vi "ElevatorSystem.vi"(5 "Motor Output":dbl, 7 "Controller Override?":bool, 8 "Scoring Deploy Status":cluster{"State":enum16{"Idle", "Deploy"}}, 9 "Scoring Heights":i32[](array[numeric]), 10 "Device Names":string[](array[string]), 11 "Intake Status":T2) -> (3 "Elevator Status":T1)   [LabVIEW 2014]
panel:
  # "Proximity Sensor"
  # "Elevator Encoder"
  # "Elevator Motor"
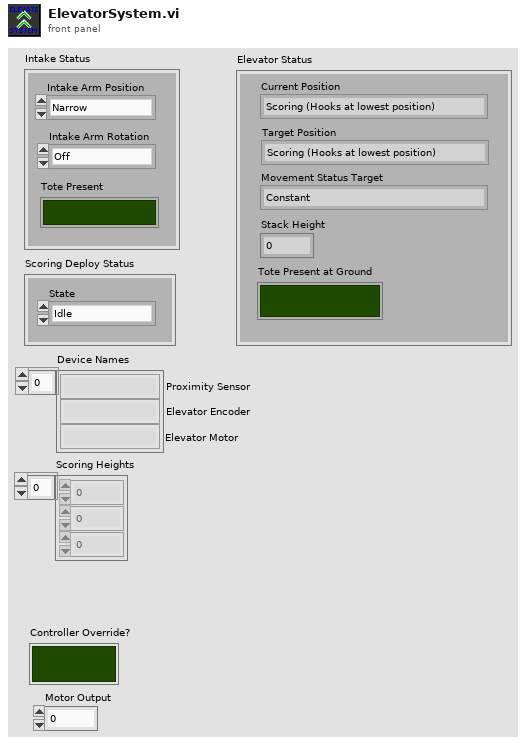
[diagram p1: front panel]
types:
  T1 = cluster{"Current Position":enum16{"Scoring (Hooks at lowest position)", "Intermediary (Between positions)", "Low (Hooks rest under lip)", "High (Holding totes up)"}, "Movement Status Target":enum16{"Constant", "Lifting", "Lowering"}, "Stack Height":i32, "Tote Present at Ground":bool, "Target Position":enum16{"Scoring (Hooks at lowest position)", "Low (Hooks rest under lip)", "High (Holding totes up)"}}
  T2 = cluster{"Intake Arm Position":enum16{"Narrow", "Wide"}, "Intake Arm Rotation":enum16{"Off", "In", "Out", "Rotate Tote"}, "Tote Present":bool}
  T3 = typedef "WPI_MotorControlDeviceRef.ctl" = cluster{"DeviceStatus":errorcluster, "Type":T4, "PWM":cluster{"Controller":T5, "PWM Channel":T6, "DeadBand":T7}, "CAN":cluster{"Device Number":u8, "Control Mode":T8, "Semaphore":T9, "Max Vout":dbl, "TalonSRX Control Mode":T10}, "Invert":bool, "TransformRef":T11, "InvTransformRef":T11}
  T4 = typedef "WPI_MotorControlType.ctl" = enum16{"PWM", "CAN", "CANTalonSRX"}
  T5 = typedef "FPGA_TypedefDigitalModule.ctl" = enum16{"Controller 1"}
  T6 = typedef "FPGA_DIOPWMChannel.ctl" = enum8{"PWM 0", "PWM 1", "PWM 2", "PWM 3", "PWM 4", "PWM 5", "PWM 6", "PWM 7", "PWM 8", "PWM 9", "PWM MXP 0", "PWM MXP 1", "PWM MXP 2", "PWM MXP 3", "PWM MXP 4", "PWM MXP 5", "PWM MXP 6", "PWM MXP 7", "PWM MXP 8", "PWM MXP 9", "Invalid"}
  T7 = typedef "WPI_PWMDeadband.ctl" = cluster{"Name":string, "maxPositivePwm":i32, "minPositivePwm":i32, "centerPwm":i32, "maxNegativePwm":i32, "minNegativePwm":i32, "angularRange":u16}
  T8 = typedef "WPI_CANJaguar_ControlMode.ctl" = enum8{"Percent VBus", "Current", "Speed", "Position", "Voltage"}
  T9 = typedef "Semaphore RefNum" = refnum<k1>
  T10 = typedef "WPI_CANTalonSRX_APIControlMode.ctl" = enum8{"Percent VBus", "Speed", "Position", "Slave", "Unchanged / Invalid"}
  T11 = typedef "WPI_PWMTransform_ConPane.ctl" = refnum<vi>
  T12 = enum16{"Scoring (Hooks at lowest position)", "Low (Hooks rest under lip)", "High (Holding totes up)"}
  T13 = cluster{"Current Position":enum16{"Scoring (Hooks at lowest position)", "Intermediary (Between positions)", "Low (Hooks rest under lip)", "High (Holding totes up)"}, "Movement Status Target":enum16{"Constant", "Lifting", "Lowering"}, "Stack Height":i32, "Tote Present at Ground":bool, "Target Position":enum16{"Scoring (Hooks at lowest position)", "Low (Hooks rest under lip)", "High (Holding totes up)", "Intermediary"}}
  T14 = enum16{"Scoring (Hooks at lowest position)", "Intermediary (Between positions)", "Low (Hooks rest under lip)", "High (Holding totes up)"}
  T15 = enum16{"Scoring (Hooks at lowest position)", "Low (Hooks rest under lip)", "High (Holding totes up)", "Intermediary"}
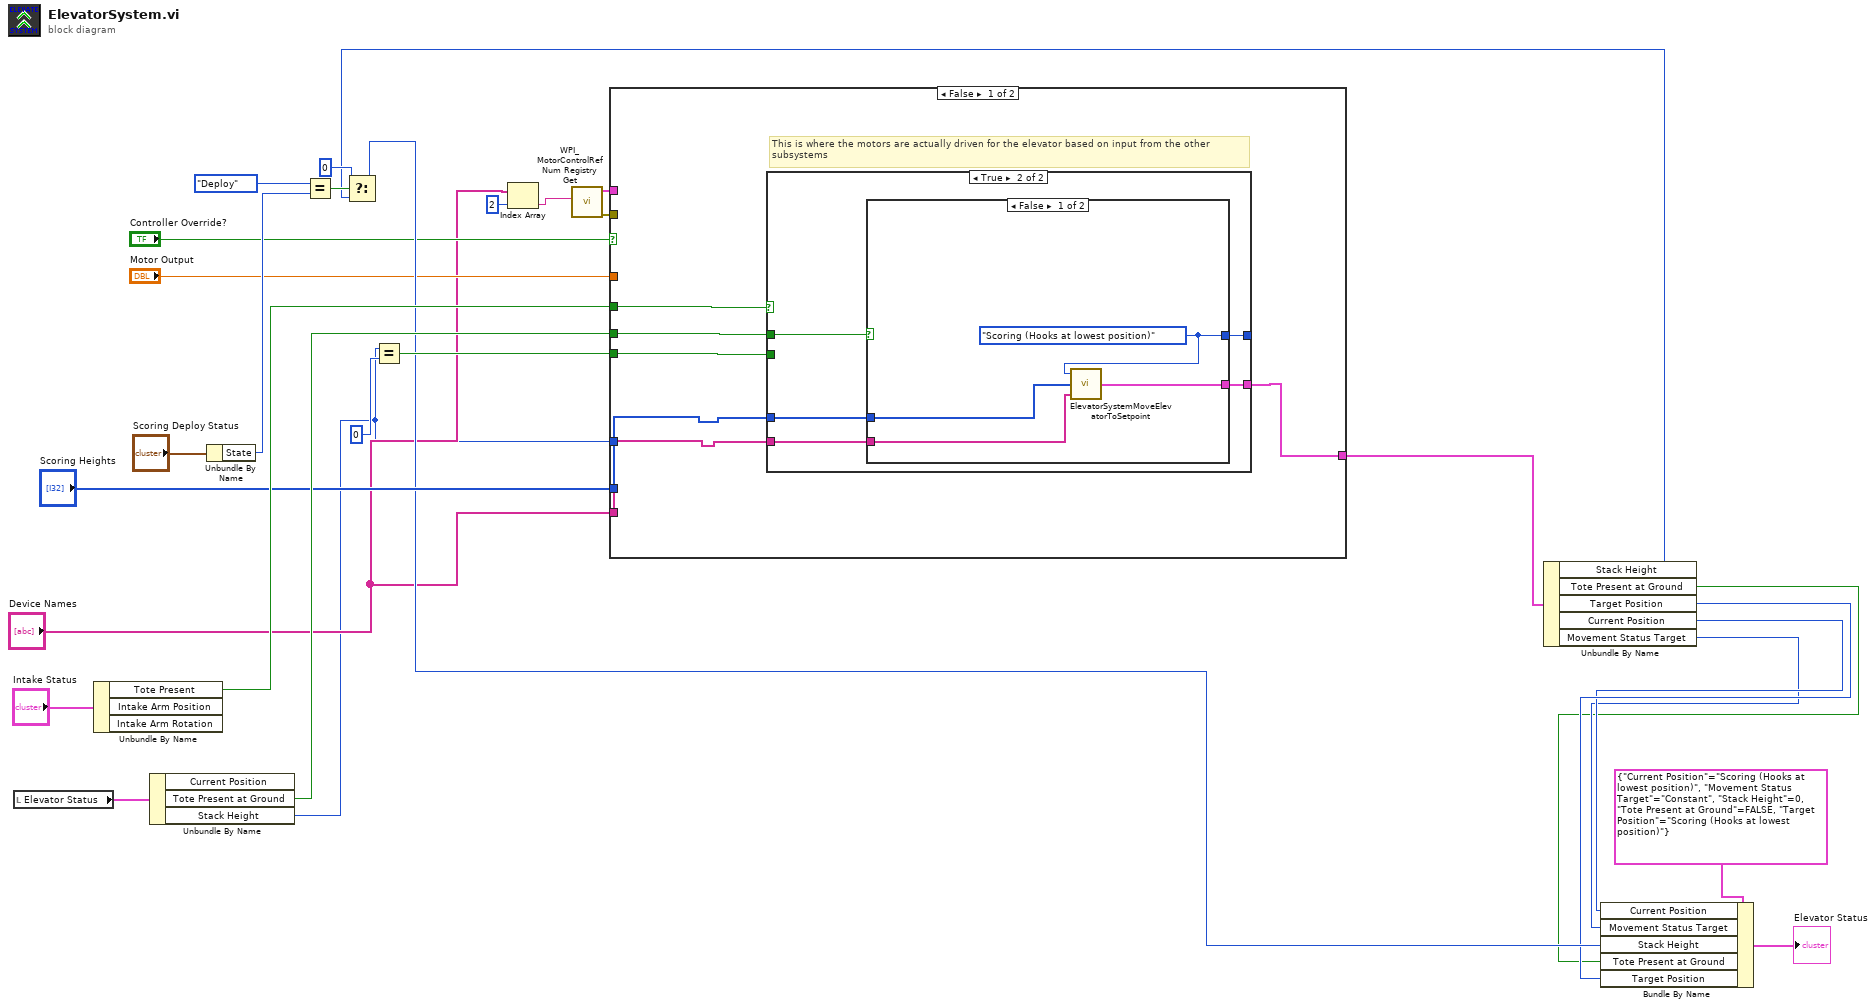
[diagram p0: block diagram]
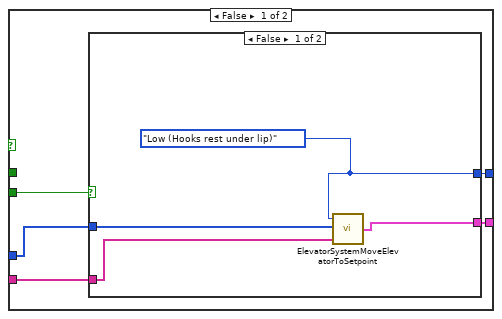
[diagram p2: hidden frame]
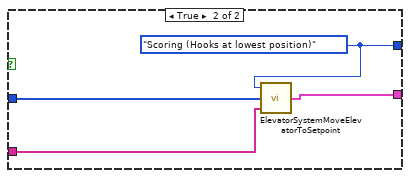
[diagram p3: hidden frame]
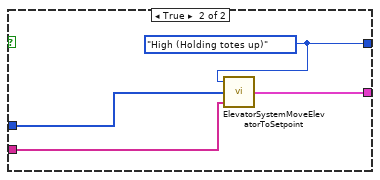
[diagram p4: hidden frame]
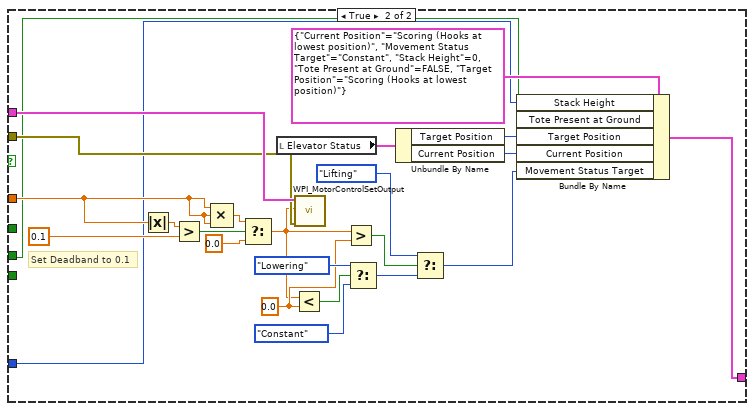
[diagram p5: hidden frame]
diagram:
  n1 = local read "Elevator Status"() -> (w28:T1)
  n2 = Unbundle By Name("Intake Status") -> ("Tote Present"=w27:bool)  [unwired: 2 out]
  n3 = Unbundle By Name(w28) -> ("Tote Present at Ground"=w17:bool, "Stack Height"=w1:i32)  [unwired: 1 out]
  n4 = Unbundle By Name("Scoring Deploy Status") -> ("State"=w23:enum16{"Idle", "Deploy"})
  n5 = Equal?(x=enum16{"Idle", "Deploy"}."Deploy", y=w23) -> (x = y?=w21:bool)
  n6 = Equal?(x=w1, y=0) -> (x = y?=w25:bool)
  n7 = Index Array(array="Device Names", index=2) -> (element=w4:string)
  n8 = call <vilib>:"WPI_MotorControlRefNum Registry Get.vi"("refnum name"=w4) -> ("error out"=w2:errorcluster, "MotorControlDevRef"=w6:T3)  [unwired: 9 in]
  n9 = case shown="False" "Controller Override?" {
    tunnel: w27 -> [w35 _]
    tunnel: w25 -> [w33 _]
    tunnel: w17 -> [w34 w62]
    tunnel: "Scoring Heights" -> [w32 _]
    tunnel: "Device Names" -> [w31 _]
    tunnel: [w30 w77] -> w15
    tunnel: "Motor Output" -> [_ w78]
    tunnel: w6 -> [_ w81]
    tunnel: w2 -> [_ w80]
    tunnel: w1 -> [_ w75]
    frame False {
      # "This is where the motors are actually driven for the elevator based on input from the other \nsubsystems"
      n10 = case shown="True" w35 {
        tunnel: w34 -> [_ w53]
        tunnel: [w39 w52] -> _
        tunnel: w33 -> [w40 _]
        tunnel: w32 -> [w38 w51]
        tunnel: w31 -> [w37 w50]
        tunnel: [w36 w49] -> w30
        frame False {
          n11 = case shown="False" w40 {
            tunnel: [w44 w48] -> w39
            tunnel: w38 -> [w43 w47]
            tunnel: w37 -> [w42 w46]
            tunnel: [w41 w45] -> w36
            frame False {
              w44 = T12."Low (Hooks rest under lip)" ("Target Position")
              n12 = call "ElevatorSystemMoveElevatorToSetpoint.vi"("Device Names"=w42, "Scoring Heights"=w43, "Target Position"=w44) -> ("Elevator Status"=w41:T13)
            }
            frame True {
              w48 = T12."Scoring (Hooks at lowest position)" ("Target Position")
              n13 = call "ElevatorSystemMoveElevatorToSetpoint.vi"("Device Names"=w46, "Scoring Heights"=w47, "Target Position"=w48) -> ("Elevator Status"=w45:T13)
            }
          }
        }
        frame True {
          n14 = case shown="False" w53 {
            tunnel: [w54 w61] -> w52
            tunnel: w51 -> [w57 w60]
            tunnel: w50 -> [w56 w59]
            tunnel: [w55 w58] -> w49
            frame False {
              w54 = T12."Scoring (Hooks at lowest position)" ("Target Position")
              n15 = call "ElevatorSystemMoveElevatorToSetpoint.vi"("Device Names"=w56, "Scoring Heights"=w57, "Target Position"=w54) -> ("Elevator Status"=w55:T13)
            }
            frame True {
              w61 = T12."High (Holding totes up)" ("Target Position")
              n16 = call "ElevatorSystemMoveElevatorToSetpoint.vi"("Device Names"=w59, "Scoring Heights"=w60, "Target Position"=w61) -> ("Elevator Status"=w58:T13)
            }
          }
        }
      }
    }
    frame True {
      w67 = 0.0 ("y")
      # "Set Deadband to 0.1"
      n17 = Absolute Value(x=w78) -> (abs(x)=w79:dbl)
      n18 = Greater?(x=w79, y=0.1) -> (0:w85:bool)
      n19 = Compound Arithmetic op=MULTIPLY(w78, w78, w78) -> (w83:dbl)
      n20 = Select(t=w83, s=w85, f=0.0) -> (s? t:f=w66:dbl)
      n21 = local read "Elevator Status"() -> (w74:T1)
      n22 = Less?(x=w66, y=w67) -> (x < y?=w64:bool)
      n23 = call <vilib>:"WPI_MotorControlSetOutput.vi"("error in (no error)"=w80, "Output"=w66, "MotorControlDevRef"=w81) -> ()  [unwired: 6 in, 3 out]
      n24 = Greater?(x=w66, y=w67) -> (0:w65:bool)
      n25 = Select(t=enum16{"Constant", "Lifting", "Lowering"}."Lowering" ("Movement Status Target"), s=w64, f=enum16{"Constant", "Lifting", "Lowering"}."Constant" ("Movement Status Target")) -> (s? t:f=w70:enum16{"Constant", "Lifting", "Lowering"})
      n26 = Unbundle By Name(w74) -> ("Target Position"=w73:T12, "Current Position"=w72:T14)
      n27 = Select(t=enum16{"Constant", "Lifting", "Lowering"}."Lifting" ("Movement Status Target"), s=w65, f=w70) -> (s? t:f=w63:enum16{"Constant", "Lifting", "Lowering"})
      n28 = Bundle By Name(cluster=T1 {"Current Position"=enum."Scoring (Hooks at lowest position)", "Movement Status Target"=enum."Constant", "Stack Height"=0, "Tote Present at Ground"=FALSE, "Target Position"=enum."Scoring (Hooks at lowest position)"} ("Elevator Status"), "Stack Height"=w75, "Tote Present at Ground"=w62, "Target Position"=w73, "Current Position"=w72, "Movement Status Target"=w63) -> (w77:T1)
    }
  }
  n29 = Unbundle By Name(w15) -> ("Stack Height"=w14:i32, "Tote Present at Ground"=w8:bool, "Target Position"=w11:T15, "Current Position"=w10:T14, "Movement Status Target"=w9:enum16{"Constant", "Lifting", "Lowering"})
  n30 = Select(t=0, s=w21, f=w14) -> (s? t:f=w13:i32)
  n31 = Bundle By Name(cluster=T1 {"Current Position"=enum."Scoring (Hooks at lowest position)", "Movement Status Target"=enum."Constant", "Stack Height"=0, "Tote Present at Ground"=FALSE, "Target Position"=enum."Scoring (Hooks at lowest position)"} ("Elevator Status 2"), "Current Position"=w10, "Movement Status Target"=w9, "Stack Height"=w13, "Tote Present at Ground"=w8, "Target Position"=w11) -> (→"Elevator Status":T1)
